vi "Climb_Teleop.vi"(2 "Joystick_Out":T1, 3 "Visited_Disabled":bool) -> ()   [LabVIEW 2018]
uses:
  Utility_VIs/Joystick_Controls.ctl
  Subsytems/Climb/Climb_Notifier.ctl
  Subsytems/Climb/Climb_Control_Type.ctl
  <vilib>/Rock Robotics/WPI/DriverStation/WPI_DriverStationRobotMode2.ctl
  Global_Variables/Robot_Global_Data.vi
  Global_Variables/Climb_Globals.vi
  Global_Variables/Sensor_Values.vi
  Global_Variables/Elevator_Globals.vi
  Global_Variables/LED_Globals.vi
  <vilib>/Rock Robotics/WPI/ThirdParty/Phoenix-LabVIEW/Motor Controller/Controls/CTRE_Phoenix_MotorControl_ControlMode.ctl
panel:
  out "Climb_Advance Climb":bool
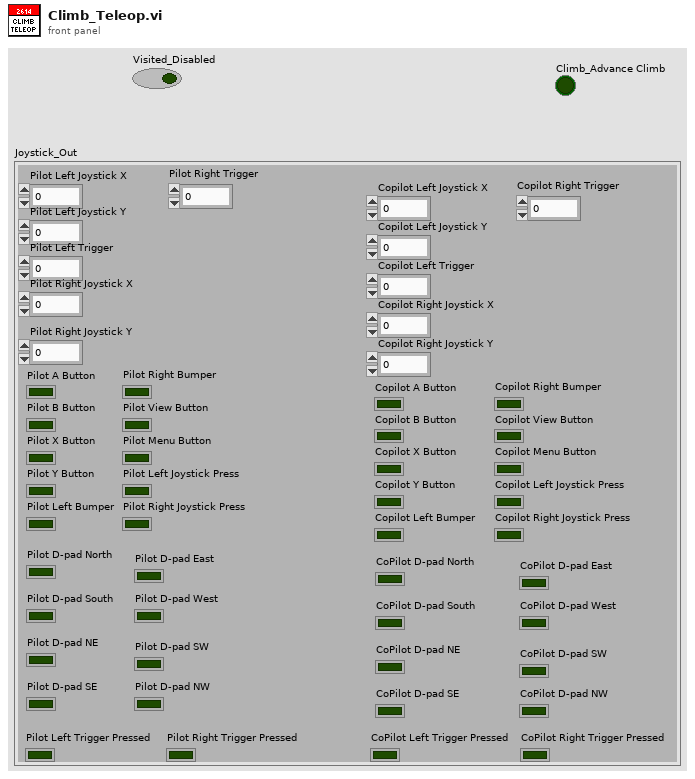
[diagram p1: front panel]
types:
  T1 = typedef "Joystick_Controls.ctl" = cluster{"Pilot Left Joystick X":dbl, "Pilot Left Joystick Y":dbl, "Pilot A Button":bool, "Pilot B Button":bool, "Pilot X Button":bool, "Pilot Y Button":bool, "Pilot Left Bumper":bool, "Pilot Right Bumper":bool, "Pilot View Button":bool, "Pilot Menu Button":bool, "Pilot Left Joystick Press":bool, "Pilot Right Joystick Press":bool, "Pilot Left Trigger":dbl, "Pilot Right Joystick X":dbl, "Pilot Right Joystick Y":dbl, "Pilot Right Trigger":dbl, "Copilot Left Joystick X":dbl, "Copilot Left Joystick Y":dbl, "Copilot A Button":bool, "Copilot B Button":bool, "Copilot X Button":bool, "Copilot Y Button":bool, "Copilot Left Bumper":bool, "Copilot Right Bumper":bool, "Copilot View Button":bool, "Copilot Menu Button":bool, "Copilot Left Joystick Press":bool, "Copilot Right Joystick Press":bool, "Copilot Left Trigger":dbl, "Copilot Right Joystick X":dbl, "Copilot Right Joystick Y":dbl, "Copilot Right Trigger":dbl, "Pilot D-pad North":bool, "Pilot D-pad South":bool, "Pilot D-pad East":bool, "Pilot D-pad West":bool, "Pilot D-pad NE ":bool, "Pilot D-pad SE":bool, "Pilot D-pad SW":bool, "Pilot D-pad NW":bool, "CoPilot D-pad North":bool, "CoPilot D-pad South":bool, "CoPilot D-pad East":bool, "CoPilot D-pad West":bool, "CoPilot D-pad NE":bool, "CoPilot D-pad SE":bool, "CoPilot D-pad SW":bool, "CoPilot D-pad NW":bool, "Pilot Left Trigger Pressed":bool, "Pilot Right Trigger Pressed":bool, "CoPilot Left Trigger Pressed":bool, "CoPilot Right Trigger Pressed":bool}
  T2 = typedef "WPI_DriverStationRobotMode2.ctl" = enum16{"Autonomous Disabled", "Autonomous Enabled", "Teleop Disabled", "Teleop Enabled", "Disconnected", "Finish", "Test Disabled", "Test Enabled", "Emergency Stopped"}
  T3 = typedef "Climb_Notifier.ctl" = cluster{"Climb_Control_Type":T4, "Brake":bool, "Manual_Climb_Up":bool, "Manual_Drive_Forward":bool, "Manual_Drive_Backward":bool, "Manual_Climb_Down":bool, "Climb_Advance":bool, "Climb_Reverse":bool, "Parameter_One":dbl, "Parameter_Two":dbl, "Parameter_Three":dbl, "Step":i32, "Climb_Notifier":refnum<notifier>, "Climb_Distance":dbl, "Level_Two":bool, "Brake_State":bool, "Toggle_Servo":bool, "Drop_Back":bool}
  T4 = typedef "Climb_Control_Type.ctl" = enum16{"No_Op", "Brake", "Manual_Climb_Up", "Manual_Climb_Down", "Manual_Drive_Forward", "Manual_Drive_Backward", "Back_Wheels_Forward", "Lift_Retract", "Lift_Extend", "Extend_to_Second_Level", "Drop_Down", "Spin"}
  T5 = typedef "CTRE_Phoenix_MotorControl_ControlMode.ctl" = u16
  T6 = typedef "WPI_MotorControlDeviceRef.ctl" = cluster{"DeviceStatus":errorcluster, "Type":T7, "PWM":cluster{"PWM Channel":T8, "DeadBand":T9}, "CAN":cluster{"Device Number":u8, "SetOutput VI Ref":variant, "GetOutput VI Ref":variant, "Enable VI Ref":variant, "Disable VI Ref":variant, "Data":variant}, "Invert":bool, "DIO PWM":cluster{"PWM \"Enable\" Channel":T8, "DIOChannel":T10, "PWM Rate":dbl}}
  T7 = typedef "WPI_MotorControlType.ctl" = enum16{"PWM", "CAN", "DIO PWM"}
  T8 = typedef "FPGA_DIOPWMChannel.ctl" = enum8{"PWM 0", "PWM 1", "PWM 2", "PWM 3", "PWM 4", "PWM 5", "PWM 6", "PWM 7", "PWM 8", "PWM 9", "PWM MXP 0", "PWM MXP 1", "PWM MXP 2", "PWM MXP 3", "PWM MXP 4", "PWM MXP 5", "PWM MXP 6", "PWM MXP 7", "PWM MXP 8", "PWM MXP 9", "Invalid"}
  T9 = typedef "WPI_PWMDeadband.ctl" = cluster{"Name":string, "maxPositivePwm":i32, "minPositivePwm":i32, "centerPwm":i32, "maxNegativePwm":i32, "minNegativePwm":i32, "angularRange":u16}
  T10 = typedef "FPGA_DIOChannel.ctl" = enum8{"DIO 0", "DIO 1", "DIO 2", "DIO 3", "DIO 4", "DIO 5", "DIO 6", "DIO 7", "DIO 8", "DIO 9", "DIO MXP 0", "DIO MXP 1", "DIO MXP 2", "DIO MXP 3", "DIO MXP 4", "DIO MXP 5", "DIO MXP 6", "DIO MXP 7", "DIO MXP 8", "DIO MXP 9", "DIO MXP 10", "DIO MXP 11", "DIO MXP 12", "DIO MXP 13", "DIO MXP 14", "DIO MXP 15", "SPI Port CS1", "SPI Port CS2", "SPI Port CS3", "SPI Port MISO", "SPI Port MOSI", "Invalid"}
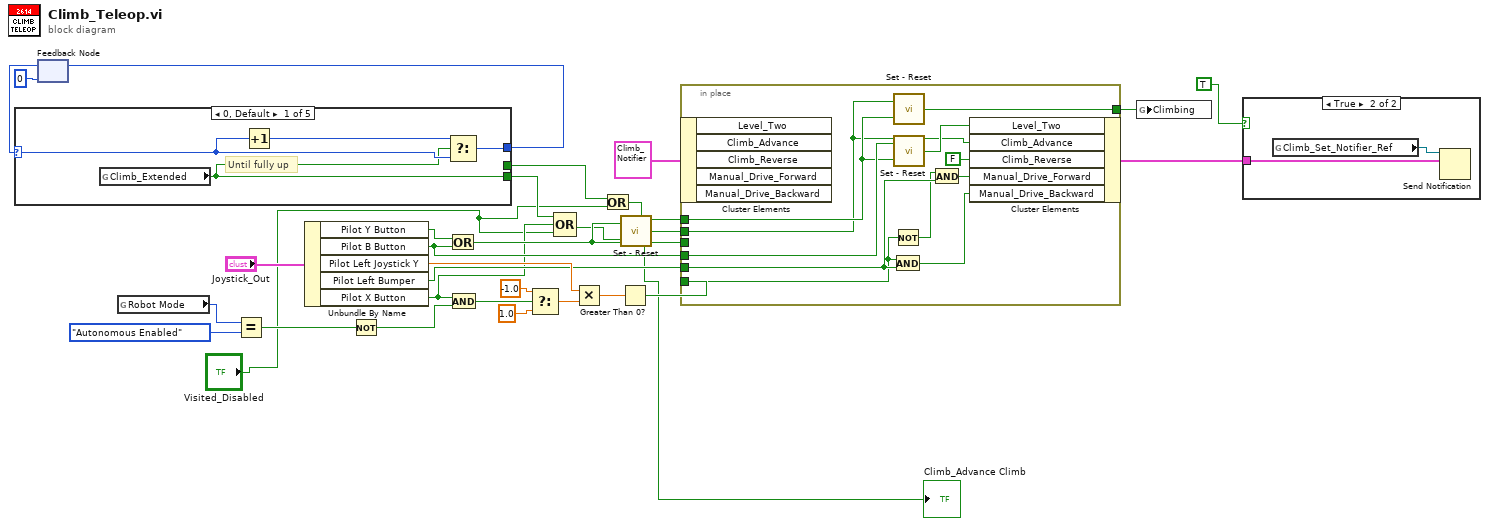
[diagram p0: block diagram]
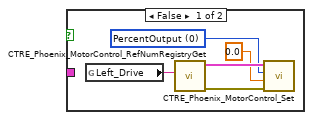
[diagram p2: hidden frame]
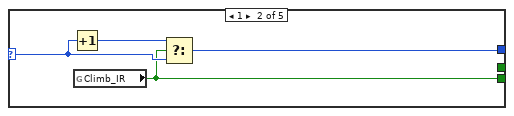
[diagram p3: hidden frame]
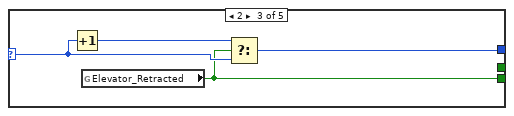
[diagram p4: hidden frame]
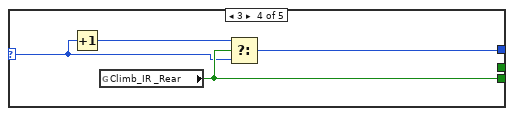
[diagram p5: hidden frame]
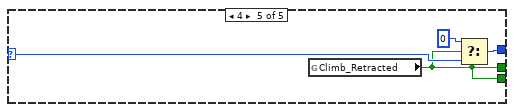
[diagram p6: hidden frame]
diagram:
  n1 = feedback #1(0) -> (w9:i32)
  n2 = case shown="0, Default" w9 {
    selector: w9 -> [w33 w36 w40 w44 w49]
    tunnel: [w32 w38 w41 w46 w50] -> w8
    tunnel: [w31 w35 w39 w45 w47] -> w7
    tunnel: [_ _ _ _ w47] -> w3
    frame 0, Default {
      # "Until fully up"
      n3 = global read "Climb_Globals.vi" "Climb_Extended"() -> (w31:bool)
      n4 = Increment(x=w33) -> (x+1=w34:i32)
      n5 = Select(t=w34, s=w31, f=w33) -> (s? t:f=w32:i32)
    }
    frame 1 {
      n6 = Increment(x=w36) -> (x+1=w37:i32)
      n7 = global read "Sensor_Values.vi" "Climb_IR"() -> (w35:bool)
      n8 = Select(t=w37, s=w35, f=w36) -> (s? t:f=w38:i32)
    }
    frame 2 {
      n9 = Increment(x=w40) -> (x+1=w42:i32)
      n10 = global read "Elevator_Globals.vi" "Elevator_Retracted"() -> (w39:bool)
      n11 = Select(t=w42, s=w39, f=w40) -> (s? t:f=w41:i32)
    }
    frame 3 {
      n12 = Increment(x=w44) -> (x+1=w43:i32)
      n13 = global read "Sensor_Values.vi" "Climb_IR _Rear"() -> (w45:bool)
      n14 = Select(t=w43, s=w45, f=w44) -> (s? t:f=w46:i32)
    }
    frame 4 {
      n15 = global read "Climb_Globals.vi" "Climb_Retracted"() -> (w47:bool)
      n16 = Select(t=0, s=w47, f=w49) -> (s? t:f=w50:i32)
    }
  }
  n17 = feedback-in #1(w8) -> ()
  n18 = global read "Robot_Global_Data.vi" "Robot Mode"() -> (w4:T2)
  n19 = Equal?(x=w4, y=WPI_DriverStationRobotMode2."Autonomous Enabled") -> (x = y?=w17:bool)
  n20 = Unbundle By Name("Joystick_Out") -> ("Pilot Y Button"=w27:bool, "Pilot B Button"=w13:bool, "Pilot Left Joystick Y"=w26:dbl, "Pilot Left Bumper"=w15:bool, "Pilot X Button"=w5:bool)
  n21 = Not(x=w17) -> (.not. x?=w16:bool)
  n22 = Or(x=w27, y=w13) -> (x .or. y?=w11:bool)
  n23 = And(x=w5, y=w16) -> (x .and. y?=w19:bool)
  n24 = Select(t=-1.0, s=w19, f=1.0) -> (s? t:f=w22:dbl)
  n25 = Compound Arithmetic op=OR(w7, w5, "Visited_Disabled") -> (w6:bool)
  n26 = Multiply(x=w26, y=w22) -> (x*y=w23:dbl)
  n27 = Or(x=w3, y="Visited_Disabled") -> (x .or. y?=w2:bool)
  n28 = Greater Than 0?(x=w23) -> (x > 0?=w25:bool)
  n29 = call "Set - Reset.vi"("Reset"=w6, "Set"=w11) -> ("Output"=w12:bool)
  "Climb_Advance Climb" <- w12
  n30 = in-place {
    in-place-border: w12 -> [w51]
    in-place-border: w11 -> [_]
    in-place-border: w13 -> [w54]
    in-place-border: w15 -> [w59]
    in-place-border: w25 -> [w58]
    in-place-border: [w56] -> w24
    in-place-border: w2 -> [w53]
    n31 = in-place-cluster #2(T3 {"Climb_Control_Type"=enum."No_Op", "Brake"=FALSE, "Manual_Climb_Up"=FALSE, "Manual_Drive_Forward"=FALSE, "Manual_Drive_Backward"=FALSE, "Manual_Climb_Down"=FALSE, "Climb_Advance"=FALSE, "Climb_Reverse"=FALSE, "Parameter_One"=0.0, "Parameter_Two"=0.0, "Parameter_Three"=0.0, "Step"=0, "Climb_Notifier"=refnum, "Climb_Distance"=0.0, "Level_Two"=FALSE, "Brake_State"=FALSE, "Toggle_Servo"=FALSE, "Drop_Back"=FALSE} ("Climb_Notifier")) -> ()  [unwired: 5 out]
    n32 = Not(x=w58) -> (.not. x?=w57:bool)
    n33 = And(x=w58, y=w59) -> (x .and. y?=w60:bool)
    n34 = call "Set - Reset.vi"("Reset"=w53, "Set"=w51) -> ("Output"=w56:bool)
    n35 = call "Set - Reset.vi"("Reset"=w53, "Set"=w54) -> ("Output"=w55:bool)
    n36 = And(x=w57, y=w59) -> (x .and. y?=w61:bool)
    n37 = in-place-cluster #2("Level_Two"=w55, "Climb_Advance"=w51, "Climb_Reverse"=FALSE, "Manual_Drive_Forward"=w61, "Manual_Drive_Backward"=w60) -> (w30:T3)
  }
  n38 = global write "LED_Globals.vi" "Climbing"(w24) -> ()
  n39 = case shown="True" TRUE {
    tunnel: w30 -> [_ w68]
    frame False {
      w62 = T5 0 items=["PercentOutput"=0, "Position"=1, "Velocity"=2, "Current"=3, "Follower"=5, "MotionProfile"=6, "MotionMagic"=7, "MotionProfileArc"=10, "Disabled"=15] ("Control Mode")
      n40 = global read "Climb_Globals.vi" "Left_Drive"() -> (w66:string)
      n41 = call <vilib>:"CTRE_Phoenix_MotorControl_RefNumRegistryGet.vi"("refnum name"=w66) -> ("error out"=w64:errorcluster, "PhoenixMotorControlDevRef"=w65:T6)  [unwired: 9 in]
      n42 = call <vilib>:"CTRE_Phoenix_MotorControl_Set.vi"("error in (no error)"=w64, "Output"=0.0, "Control Mode"=w62, "PhoenixMotorControlDevRef"=w65) -> ()  [unwired: 6 in, 2 out]
    }
    frame True {
      n43 = global read "Climb_Globals.vi" "Climb_Set_Notifier_Ref"() -> (w67:refnum<notifier>)
      n44 = Send Notification(notification=w68, notifier=w67) -> ()  [unwired: 1 in, 2 out]
    }
  }
